vi "Edit Panel Example.vi"() -> ()   [LabVIEW 2015]
uses:
  myPanel/Panel Control_Ref/Panel Controller.lvclass
  myPanel/GUI/GUI Controls/Button_UI/Private/Button_UI(Classic).ctl
  myPanel/Panel Control/Panel Data/Type Definition/Panel Controls and VI Refnum.ctl
  myPanel/GUI/GUI Builder Director/GUI Control Builder Director.lvclass
  EditPanel_class/EditPanel API.lvclass/EditPanel API.ctl
  myPanel/GUI/GUI Builder Director/GUI Control Builder Director.lvclass/GUI Control Builder Director.ctl
  myPanel/Panel to Console Behaviors/Delete Control In Panel/Delete Control_Behavior.lvclass
  myPanel/Panel to Console Behaviors/Delete Control In Panel/Delete Control_Behavior.lvclass/Delete Control_Behavior.ctl
  Panel Control_Interface/Panel_interface/Panel Controller Interface.lvclass
  EditPanel_class/EditPanel API.lvclass
  myPanel/GUI/GUI Controls/Button_UI/Button_UI.lvclass
panel:
  in  "Pane(Class_Refnum)":refnum<class "Panel Controller.lvclass">
  in  "UI_UnEditable":bool
  in  "UI_Editable":bool
  in  "UI_Delete":bool
  in  "UI_Add":bool
  in  "sdfgf":T1
  in  "OK Button":bool
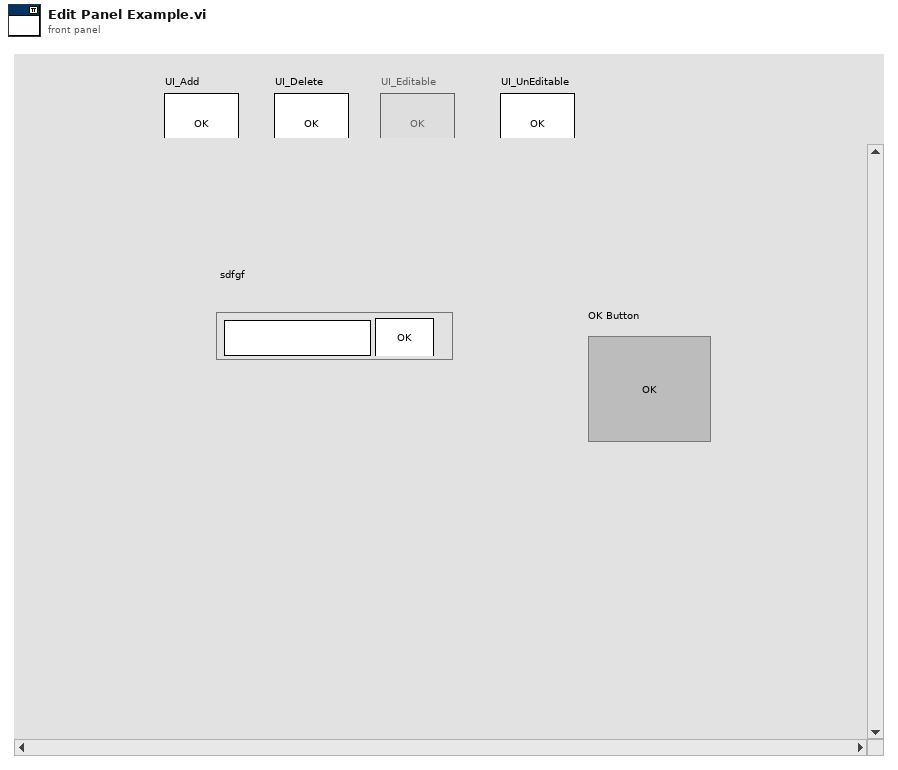
[diagram p1: front panel]
types:
  T1 = typedef "Button_UI.lvclass/Button_UI(Classic).ctl" = cluster{"Protocol":string, "Push":bool}
  T2 = typedef "Panel Controller.lvclass/Panel Controls and VI Refnum.ctl" = cluster{"UI_UnEditable":refnum<vi>, "UI_Editable":refnum<vi>, "UI_Delete":refnum<vi>, "UI_Add":refnum<vi>, "This VI":refnum<vi>}
  T3 = typedef "eventvkey.ctl" = enum16{"ASCII", "Enter", "Return", "Shift", "Ctrl", "Alt", "Cmd", "Opt", "Caps", "NumLock", "Clear", "Break", "Up", "Down", "Left", "Right", "Insert", "Delete", "Home", "End", "PageUp", "PageDown", "Escape", "Help", "Pause", "ScrollLock", "F1", "F2", "F3", "F4", "F5", "F6", "F7", "F8", "F9", "F10", "F11", "F12", "F13", "F14", "F15", "F16", "F17", "F18", "F19", "F20", "F21", "F22", "F23", "F24", "Play", "VolumeUp", "VolumeDown", "Mute", "Two Byte Char"}
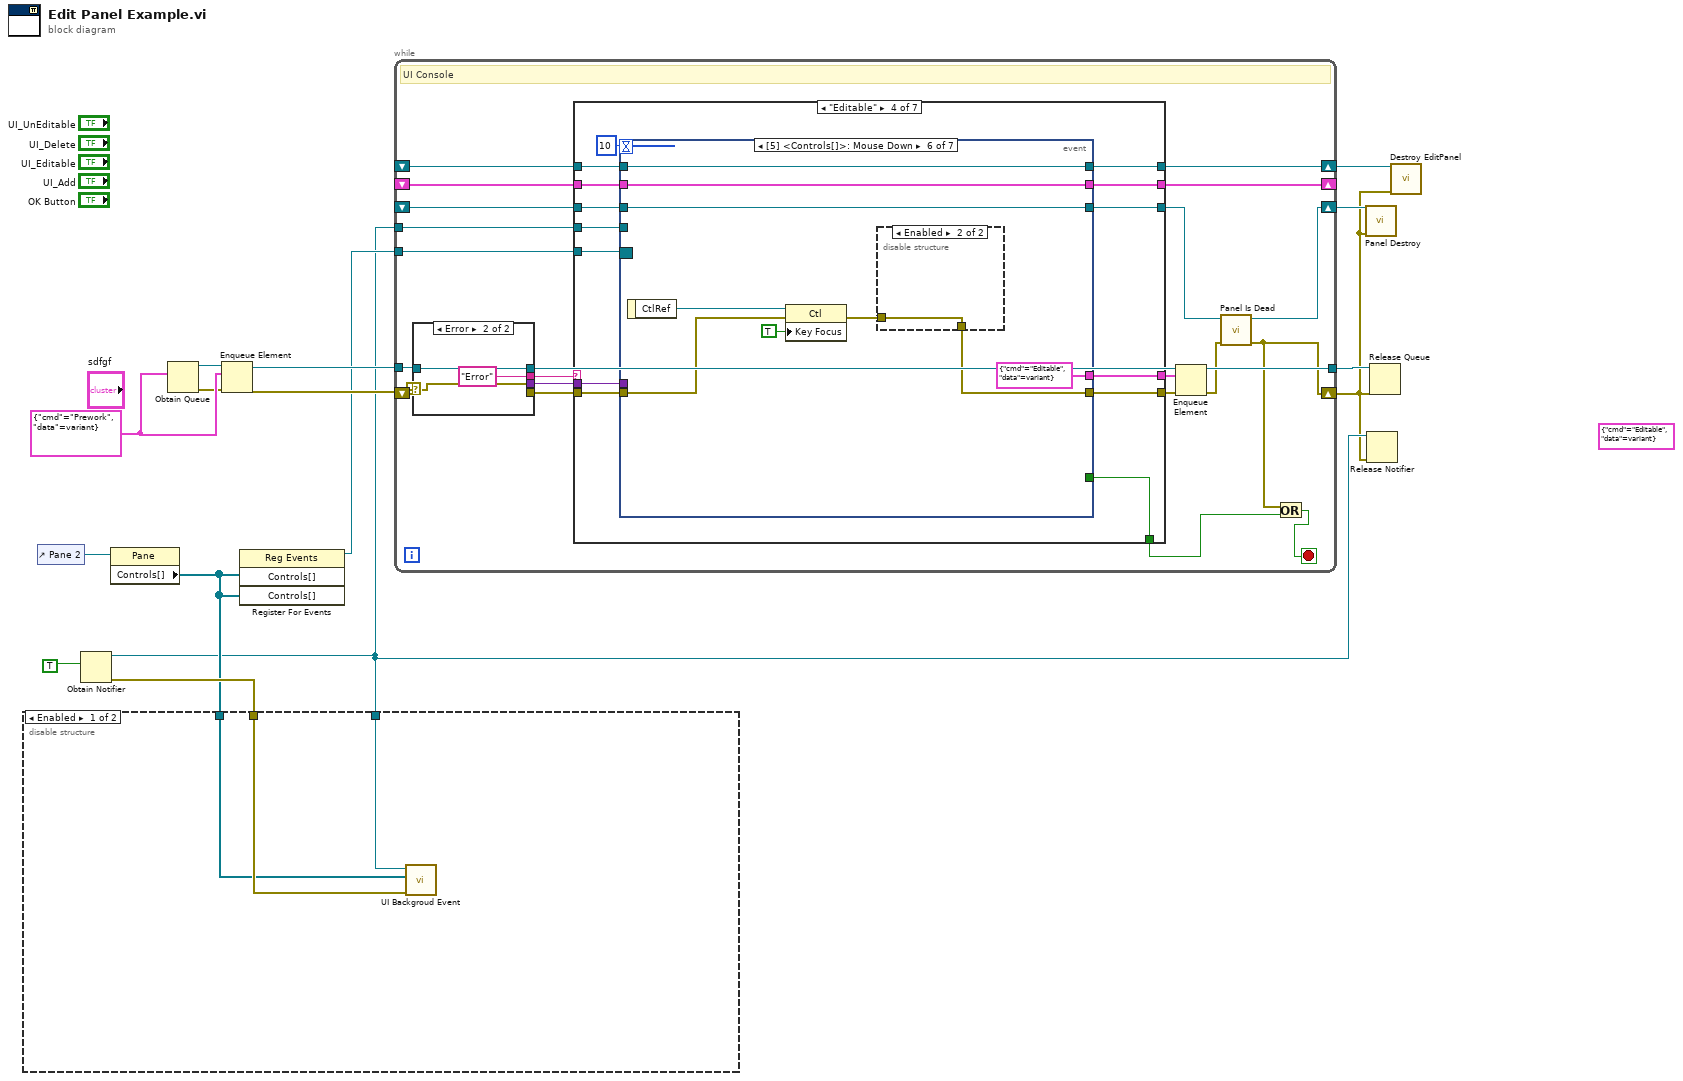
[diagram p0: block diagram]
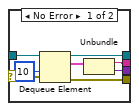
[diagram p3: hidden frame]
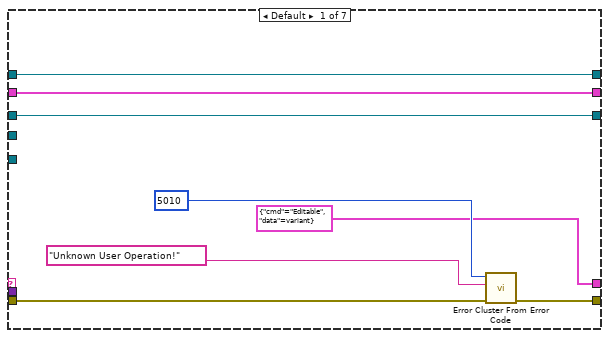
[diagram p4: hidden frame]
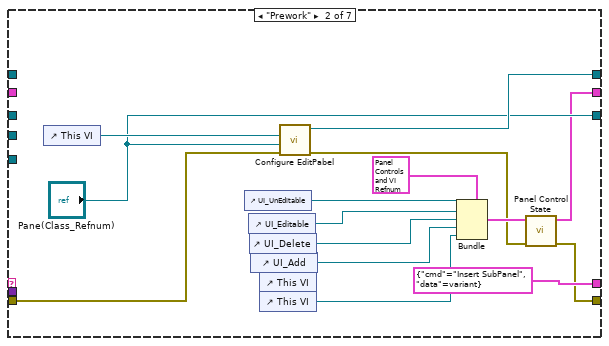
[diagram p5: hidden frame]
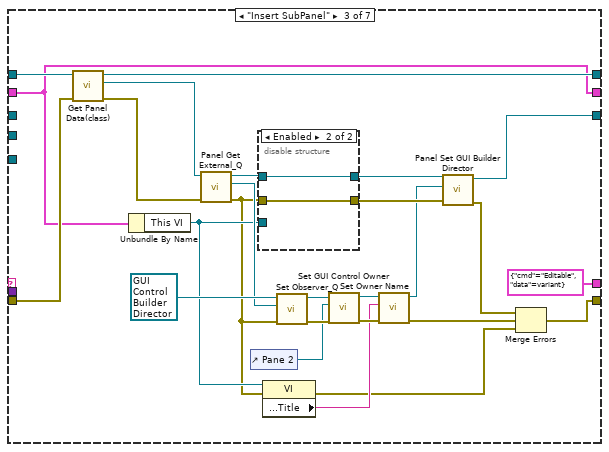
[diagram p6: hidden frame]
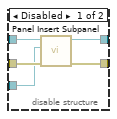
[diagram p7: hidden frame]
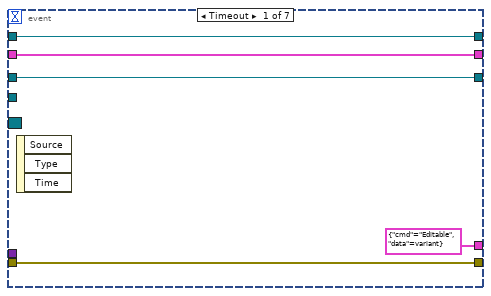
[diagram p8: hidden frame]
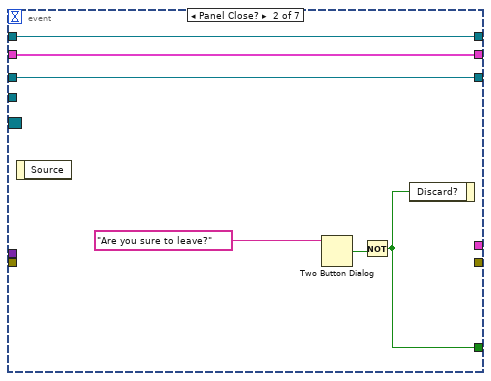
[diagram p9: hidden frame]
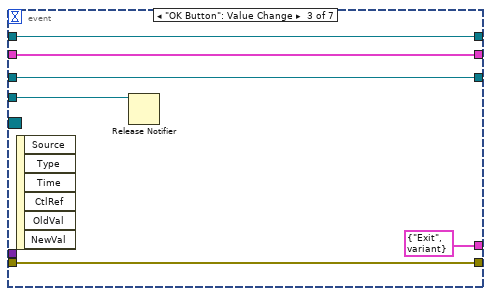
[diagram p10: hidden frame]
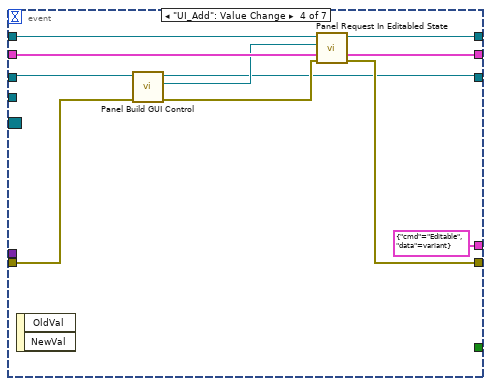
[diagram p11: hidden frame]
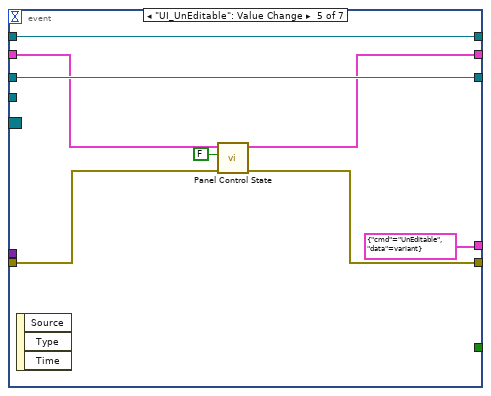
[diagram p12: hidden frame]
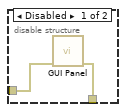
[diagram p13: hidden frame]
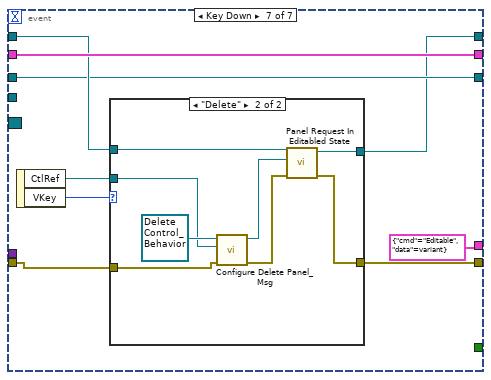
[diagram p14: hidden frame]
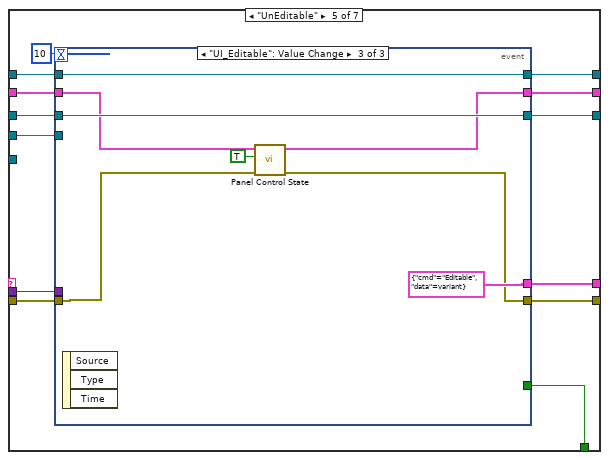
[diagram p16: hidden frame]
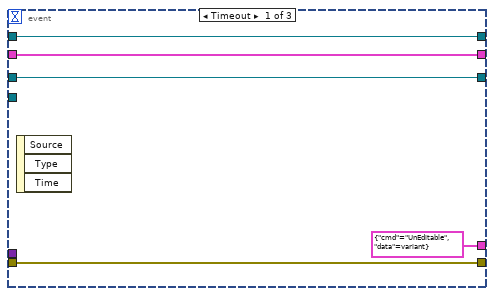
[diagram p17: hidden frame]
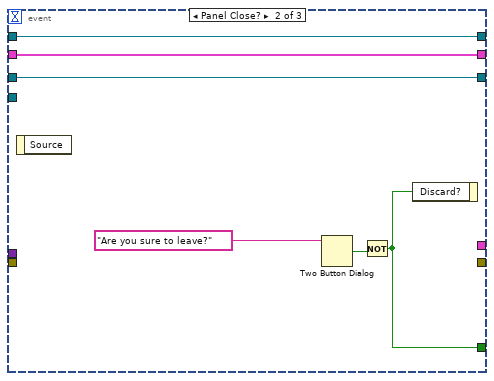
[diagram p18: hidden frame]
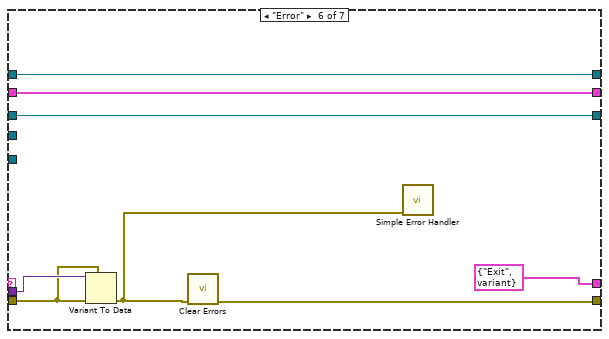
[diagram p19: hidden frame]
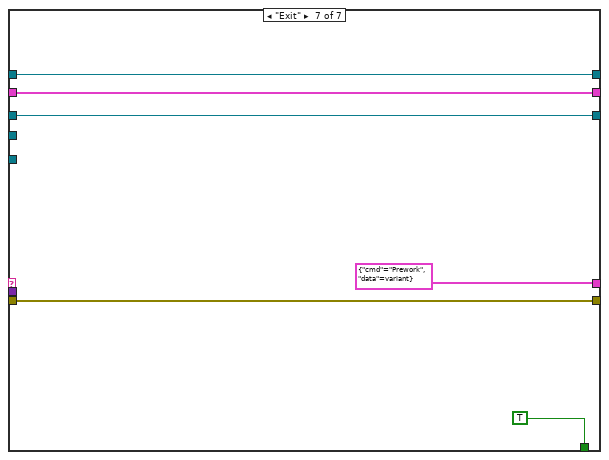
[diagram p20: hidden frame]
diagram:
  (unwired) cluster{"cmd":string, "data":variant} {"cmd"="Editable", "data"=variant}
  w12 = cluster{"cmd":string, "data":variant} {"cmd"="Prework", "data"=variant}
  n1 = control-ref of="Pane 2"() -> (w5:refnum<vi>)
  n2 = Obtain Notifier(notification data type=TRUE) -> (notifier out=w2:refnum<notifier>, error out=w15:errorcluster)  [unwired: 3 in, 1 out]
  n3 = property class="Pane"(reference=w5) -> ("Controls[]"=w4:refnum<vi>[])  [unwired: 1 in, 2 out]
  n4 = disable-structure shown="Enabled" {
    disable-tunnel: w15 -> [w17 _]
    disable-tunnel: w2 -> [w18 _]
    disable-tunnel: w4 -> [w16 _]
    frame Enabled {
      n5 = call "UI Backgroud Event.vi"("error in (no error)"=w17, "Controls[]"=w16, "Notifier"=w18) -> ()  [unwired: 8 in, 1 out]
    }
    frame Disabled {
    }
  }
  n6 = Obtain Queue(element data type=w12) -> (queue out=w8:refnum<queue>, error out=w9:errorcluster)  [unwired: 4 in, 1 out]
  n7 = Enqueue Element(queue=w8, element=w12, error in (no error)=w9) -> (queue out=w10:refnum<queue>, error out=w11:errorcluster)  [unwired: 1 in, 1 out]
  n8 = register-events(w4, w4) -> (reference out=w3:refnum<event-registration>)  [unwired: 2 in, 1 out]
  n9 = while {
    tunnel: w10 -> [w39]
    tunnel: [w25] -> w13
    shift-right: [w21] -> w1
    shift-left: w11 -> [w40]
    tunnel: w2 -> [w32]
    shift-right: [w31] -> w7
    shift-left: _ -> [w30]
    shift-right: [w23] -> w6
    shift-left: _ -> [w29]
    shift-right: [w28] -> _
    shift-left: _ -> [w27]
    tunnel: w3 -> [w26]
    stop <- w19 stop-if-true
    # "UI Console"
    n10 = case shown="Error" w40 {
      selector: w40 -> [w47 w50]
      tunnel: w39 -> [w48 w51]
      tunnel: [w45 w51] -> w37
      tunnel: [w44 _] -> w35
      tunnel: [w42 "Error" ("cmd")] -> w36
      tunnel: [w41 w50] -> w38
      frame No Error {
        n11 = Dequeue Element(queue=w48, timeout in ms (-1)=10, error in (no error)=w47) -> (queue out=w45:refnum<queue>, element=w43:cluster{"cmd":string, "data":variant}, error out=w44:errorcluster)  [unwired: 1 out]
        n12 = Unbundle(w43) -> ("cmd"=w42:string, "data"=w41:variant)
      }
      frame Error {
      }
    }
    n13 = case shown="\"Editable\"" w36 {
      tunnel: w38 -> [_ _ _ w121 w200 w227 _]
      tunnel: w35 -> [w56 w72 w99 w120 w199 w226 w228]
      tunnel: [cluster{"cmd":string, "data":variant} {"cmd"="Editable", "data"=variant} cluster{"cmd":string, "data":variant} {"cmd"="Insert SubPanel", "data"=variant} cluster{"cmd":string, "data":variant} {"cmd"="Editable", "data"=variant} w118 w197 cluster{"cmd":string, "data":variant} {"cmd"="Exit", "data"=variant} cluster{"cmd":string, "data":variant} {"cmd"="Prework", "data"=variant}] -> w34
      tunnel: [w57 w60 w83 w116 w195 w220 w228] -> w33
      tunnel: [_ _ _ w117 w196 _ TRUE] -> w20
      tunnel: w32 -> [_ _ _ w113 w192 _ _]
      tunnel: [w53 w71 w98 w111 w190 w223 w230] -> w31
      tunnel: w30 -> [w53 _ w100 w115 w194 w223 w230]
      tunnel: [w54 "Pane(Class_Refnum)" w93 w112 w191 w224 w231] -> w24
      tunnel: w29 -> [w54 _ _ w114 w193 w224 w231]
      tunnel: [w52 w62 w96 w109 w188 w222 w229] -> w28
      tunnel: w27 -> [w52 _ w96 w110 w189 w222 w229]
      tunnel: w26 -> [_ _ _ w108 _ _ _]
      frame Default {
        n14 = call <vilib>:"Error Cluster From Error Code.vi"("error in (no error)"=w56, "error message (\"\")"="Unknown User Operation!" ("error message (\"\")"), "error code (0)"=5010) -> ("error out"=w57:errorcluster)  [unwired: 6 in]
      }
      frame "Prework" {
        n15 = control-ref of="This VI"() -> (w73:refnum<vi>)
        n16 = control-ref of="UI_UnEditable"() -> (w69:refnum<vi>)
        n17 = control-ref of="UI_Editable"() -> (w68:refnum<vi>)
        n18 = control-ref of="UI_Delete"() -> (w67:refnum<vi>)
        n19 = control-ref of="UI_Add"() -> (w66:refnum<vi>)
        n20 = control-ref of="This VI"() -> ()  [unwired: 1 out]
        n21 = control-ref of="This VI"() -> (w65:refnum<vi>)
        n22 = call "Configure EditPabel.vi"("error in (no error)"=w72, "Panel"="Pane(Class_Refnum)", "vi reference"=w73) -> ("error out"=w61:errorcluster, "EditPanel out"=w71:refnum<class "EditPanel API.lvclass">)  [unwired: 7 in]
        n23 = Bundle(cluster=T2 {"UI_UnEditable"=refnum, "UI_Editable"=refnum, "UI_Delete"=refnum, "UI_Add"=refnum, "This VI"=refnum}, "UI_UnEditable"=w69, "UI_Editable"=w68, "UI_Delete"=w67, "UI_Add"=w66, "This VI"=w65) -> (w63:T2)
        n24 = call "Panel Control State.vi"("error in (no error)"=w61, "Panel Controls and VI Refnum"=w63) -> ("error out"=w60:errorcluster, "Panel Controls and VI Refnum out"=w62:T2)  [unwired: 8 in]
      }
      frame "Insert SubPanel" {
        n25 = call "Get Panel Data(class).vi"("error in (no error)"=w99, "EditPanel API in"=w100) -> ("error out"=w87:errorcluster, "Panel"=w90:refnum<class "Panel Controller Interface.lvclass">, "EditPanel API out"=w98:refnum<class "EditPanel API.lvclass">)  [unwired: 7 in]
        n26 = Unbundle By Name(w96) -> ("This VI"=w78:refnum<vi>)
        n27 = call-dynamic "Panel Get External_Q.vi"("error in (no error)"=w87, "Panel in"=w90) -> ("error out"=w76:errorcluster, "External_Q"=w88:refnum<class "Message Enqueuer.lvclass">, "Panel out"=w89:refnum<class "Panel Controller Interface.lvclass">)  [unwired: 7 in]
        n28 = control-ref of="Pane 2"() -> (w85:refnum<vi>)
        n29 = disable-structure shown="Enabled" {
          disable-tunnel: w89 -> [w105 w107]
          disable-tunnel: w76 -> [w104 w106]
          disable-tunnel: [w103 w107] -> w95
          disable-tunnel: [w102 w106] -> w94
          disable-tunnel: w78 -> [w101 _]
          frame Disabled {
            n30 = call-dynamic "Panel Insert Subpanel.vi"("error in (no error)"=w104, "VI Refnum"=w101, "Panel in"=w105) -> ("error out"=w102:errorcluster, "Panel out"=w103:refnum<class "Panel Controller Interface.lvclass">)  [unwired: 7 in]
          }
          frame Enabled {
          }
        }
        n31 = property class="VI"(reference=w78, error in=w76) -> (error out=w75:errorcluster, "Front Panel.Title"=w77:string)  [unwired: 1 out]
        n32 = call "Set Observer_Q.vi"("error in (no error)"=w76, "Observer Q"=w88, "GUI Control Builder Director in"=refnum<class "GUI Control Builder Director.lvclass"> refnum) -> ("error out"=w86:errorcluster, "GUI Control Builder Director out"=w92:refnum<class "GUI Control Builder Director.lvclass">)  [unwired: 7 in]
        n33 = call "Set GUI Control Owner.vi"("error in (no error)"=w86, "GUI Control Owner"=w85, "GUI Control Builder Director in"=w92) -> ("error out"=w81:errorcluster, "GUI Control Builder Director out"=w82:refnum<class "GUI Control Builder Director.lvclass">)  [unwired: 7 in]
        n34 = call "Set Owner Name.vi"("error in (no error)"=w81, "Owner Name"=w77, "GUI Control Builder Director in"=w82) -> ("error out"=w79:errorcluster, "GUI Control Builder Director out"=w80:refnum<class "GUI Control Builder Director.lvclass">)  [unwired: 7 in]
        n35 = call-dynamic "Panel Set GUI Builder Director.vi"("error in (no error)"=w94, "GUI Control Builder Director.lvclass"=w80, "Panel in"=w95) -> ("error out"=w84:errorcluster, "Panel out"=w93:refnum<class "Panel Controller Interface.lvclass">)  [unwired: 7 in]
        n36 = Merge Errors(w84, w79, w75) -> (w83:errorcluster)
      }
      frame "Editable" {
        n37 = event shown="[5] <Controls[]>: Mouse Down" {
          selector: w108 -> [_ _ _ _ _ _ _]
          dyn-events: _ -> [_ _ _ _ _ _ _]
          timeout: 10 -> [_ _ _ _ _ _ _]
          tunnel: w121 -> [_ _ _ _ _ _ _]
          tunnel: w120 -> [w125 _ w134 w139 w152 w161 w173]
          tunnel: [cluster{"cmd":string, "data":variant} {"cmd"="Editable", "data"=variant} _ cluster{"cmd":string, "data":variant} {"cmd"="Exit", "data"=variant} cluster{"cmd":string, "data":variant} {"cmd"="Editable", "data"=variant} cluster{"cmd":string, "data":variant} {"cmd"="UnEditable", "data"=variant} cluster{"cmd":string, "data":variant} {"cmd"="Editable", "data"=variant} cluster{"cmd":string, "data":variant} {"cmd"="Editable", "data"=variant}] -> w118
          tunnel: [_ w130 _ _ _ _ _] -> w117
          tunnel: [w125 _ w134 w147 w151 w157 w170] -> w116
          tunnel: w115 -> [w124 w129 w138 w148 w155 w164 w174]
          tunnel: w114 -> [w123 w128 w136 w143 w156 w165 w172]
          tunnel: w113 -> [_ _ w137 _ _ _ _]
          tunnel: [w123 w128 w136 w140 w156 w165 w172] -> w112
          tunnel: [w124 w129 w138 w146 w155 w164 w171] -> w111
          tunnel: w110 -> [w122 w127 w133 w144 w153 w163 w177]
          tunnel: [w122 w127 w133 w144 w150 w163 w177] -> w109
          event Timeout {
            n38 = event-data() -> ()  [unwired: 1 in, 3 out]
          }
          event Panel Close? {
            n39 = event-data() -> ()  [unwired: 1 in, 1 out]
            n40 = Two Button Dialog(message="Are you sure to leave?") -> (T button?=w131:bool)  [unwired: 2 in]
            n41 = Not(x=w131) -> (.not. x?=w130:bool)
            n42 = event-data("Discard?"=w130) -> ()  [unwired: 1 in, 1 out]
          }
          event "OK Button": Value Change {
            n43 = event-data() -> ()  [unwired: 1 in, 6 out]
            n44 = Release Notifier(notifier=w137) -> ()  [unwired: 2 in, 3 out]
          }
          event "UI_Add": Value Change {
            n45 = event-data() -> ()  [unwired: 1 in, 2 out]
            n46 = call-dynamic "Panel Build GUI Control.vi"("error in (no error)"=w139, "Panel in"=w143) -> ("error out"=w141:errorcluster, "Panel Behavior"=w142:refnum<class "Panel Behavior.lvclass">, "Panel out"=w140:refnum<class "Panel Controller Interface.lvclass">)  [unwired: 7 in]
            n47 = call "Panel Request In Editabled State.vi"("error in (no error)"=w141, "Panel Behavior(class)"=w142, "EditPanel in"=w148) -> ("error out"=w147:errorcluster, "EditPanel out"=w146:refnum<class "EditPanel API.lvclass">)  [unwired: 7 in]
          }
          event "UI_UnEditable": Value Change {
            n48 = event-data() -> ()  [unwired: 1 in, 3 out]
            n49 = call "Panel Control State.vi"("error in (no error)"=w152, "Editable(True)"=FALSE, "Panel Controls and VI Refnum"=w153) -> ("error out"=w151:errorcluster, "Panel Controls and VI Refnum out"=w150:T2)  [unwired: 7 in]
          }
          event Mouse Down {
            n50 = event-data() -> ("CtlRef"=w162:refnum<vi>)  [unwired: 1 in]
            n51 = property class="Ctl"(reference=w162, error in=w161, "Key Focus"=TRUE) -> (error out=w158:errorcluster)  [unwired: 1 out]
            n52 = disable-structure shown="Enabled" {
              disable-tunnel: w158 -> [w167 w168]
              disable-tunnel: [w166 w168] -> w157
              frame Disabled {
                n53 = call "GUI Panel.vi"("error in (no error)"=w167) -> ("error out"=w166:errorcluster)  [unwired: 10 in]
              }
              frame Enabled {
              }
            }
          }
          event Key Down {
            n54 = event-data() -> ("CtlRef"=w175:refnum<vi>, "VKey"=w176:T3)  [unwired: 1 in]
            n55 = case shown="\"Delete\"" w176 {
              tunnel: w175 -> [_ w186]
              tunnel: w174 -> [w179 w184]
              tunnel: w173 -> [w178 w185]
              tunnel: [w179 w181] -> w171
              tunnel: [w178 w180] -> w170
              frame Default {
              }
              frame "Delete" {
                n56 = call "Configure Delete Panel_Msg.vi"("error in (no error)"=w185, "Ctl Ref"=w186, "Delete Panel Control_Msg"=refnum<class "Delete Control_Behavior.lvclass"> refnum ("Delete Control In Panel_Msg")) -> ("error out"=w182:errorcluster, "Delete Panel Control_Msg"=w183:refnum<class "Delete Control_Behavior.lvclass">)  [unwired: 7 in]
                n57 = call "Panel Request In Editabled State.vi"("error in (no error)"=w182, "Panel Behavior(class)"=w183, "EditPanel in"=w184) -> ("error out"=w180:errorcluster, "EditPanel out"=w181:refnum<class "EditPanel API.lvclass">)  [unwired: 7 in]
              }
            }
          }
        }
      }
      frame "UnEditable" {
        n58 = event shown="[2] \"UI_Editable\": Value Change" {
          selector: _ -> [_ _ _]
          dyn-events: _ -> [_ _ _]
          timeout: 10 -> [_ _ _]
          tunnel: w200 -> [_ _ _]
          tunnel: w199 -> [w204 _ w214]
          tunnel: [cluster{"cmd":string, "data":variant} {"cmd"="UnEditable", "data"=variant} _ cluster{"cmd":string, "data":variant} {"cmd"="Editable", "data"=variant}] -> w197
          tunnel: [_ w209 _] -> w196
          tunnel: [w204 _ w213] -> w195
          tunnel: w194 -> [w203 w208 w218]
          tunnel: w193 -> [w202 w207 w219]
          tunnel: w192 -> [_ _ _]
          tunnel: [w202 w207 w219] -> w191
          tunnel: [w203 w208 w218] -> w190
          tunnel: w189 -> [w201 w206 w216]
          tunnel: [w201 w206 w215] -> w188
          event Timeout {
            n59 = event-data() -> ()  [unwired: 1 in, 3 out]
          }
          event Panel Close? {
            n60 = event-data() -> ()  [unwired: 1 in, 1 out]
            n61 = Two Button Dialog(message="Are you sure to leave?") -> (T button?=w210:bool)  [unwired: 2 in]
            n62 = Not(x=w210) -> (.not. x?=w209:bool)
            n63 = event-data("Discard?"=w209) -> ()  [unwired: 1 in, 1 out]
          }
          event "UI_Editable": Value Change {
            n64 = event-data() -> ()  [unwired: 1 in, 3 out]
            n65 = call "Panel Control State.vi"("error in (no error)"=w214, "Editable(True)"=TRUE, "Panel Controls and VI Refnum"=w216) -> ("error out"=w213:errorcluster, "Panel Controls and VI Refnum out"=w215:T2)  [unwired: 7 in]
          }
        }
      }
      frame "Error" {
        n66 = Variant To Data(error in=w226, type=w226, Variant=w227) -> (error out=w221:errorcluster)  [unwired: 1 out]
        n67 = call <vilib>:"Clear Errors.vi"("error in (no error)"=w221) -> ("error out"=w220:errorcluster)  [unwired: 5 in, 1 out]
        n68 = call <vilib>:"Simple Error Handler.vi"("error in (no error)"=w221) -> ()  [unwired: 4 in, 5 out]
      }
      frame "Exit" {
      }
    }
    n69 = Enqueue Element(queue=w37, element=w34, error in (no error)=w33) -> (queue out=w25:refnum<queue>, error out=w22:errorcluster)  [unwired: 1 in, 1 out]
    n70 = call-dynamic "Panel Is Dead.vi"("error in (no error)"=w22, "Panel in"=w24) -> ("error out"=w21:errorcluster, "Panel out"=w23:refnum<class "Panel Controller Interface.lvclass">)  [unwired: 8 in]
    n71 = Or(x=w21, y=w20) -> (x .or. y?=w19:bool)
  }
  n72 = call-dynamic "Panel Destroy.vi"("error in (no error)"=w1, "Panel in"=w6) -> ()  [unwired: 8 in, 2 out]
  n73 = Release Notifier(notifier=w2, error in (no error)=w1) -> ()  [unwired: 1 in, 3 out]
  n74 = Release Queue(queue=w13, error in (no error)=w1) -> ()  [unwired: 1 in, 3 out]
  n75 = call "Destroy EditPanel.vi"("error in (no error)"=w1, "EditPanel in"=w7) -> ()  [unwired: 8 in, 2 out]
